vi "FL_Decode_RAW_to_DEC_bit_split_2b.vi"(2 "Read buffer text to decode":string, 3 "Input timestamp":timestamp, 4 "SB size (loc. var. only)":u8) -> (0 "DEC output cluster":T1)   [LabVIEW 2018, in "Tracker.lvlib"]
uses:
  Tracker.lvlib
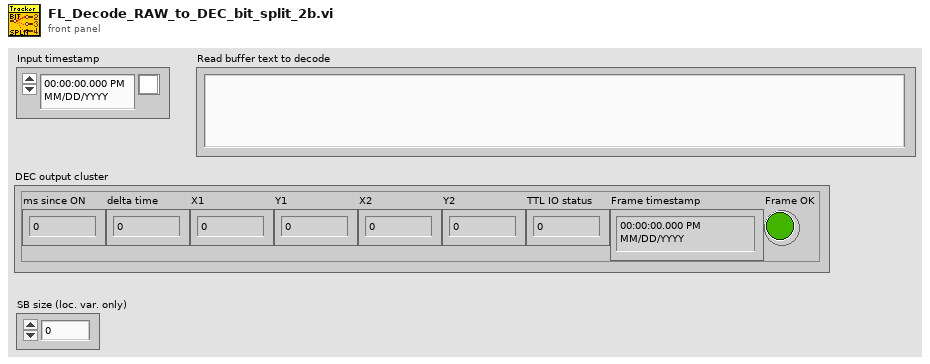
[diagram p1: front panel]
types:
  T1 = cluster{"ms since ON":u32, "delta time":u32, "X1":sgl, "Y1":sgl, "X2":sgl, "Y2":sgl, "TTL IO status":u8, "Frame timestamp":timestamp, "Frame OK":bool}
  T2 = cluster{"Half-width of the sensor board":sgl, "Half-height of the sensor board":sgl, "Sensors grid step":sgl}
  T3 = cluster{u32, u32, sgl, sgl, sgl, sgl, u8, "Input timestamp":timestamp, bool}
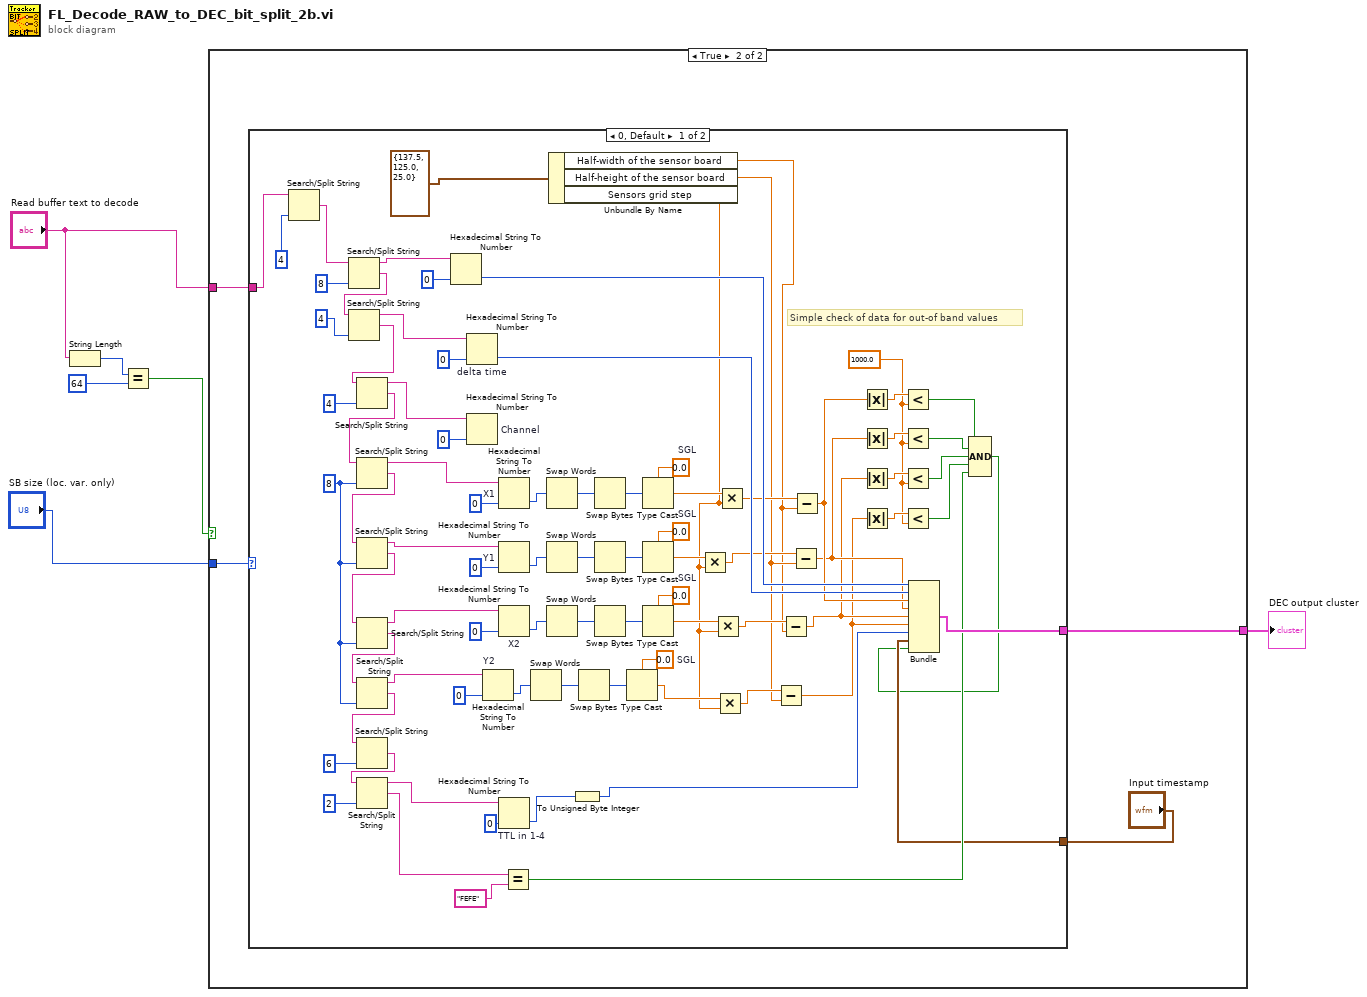
[diagram p0: block diagram]
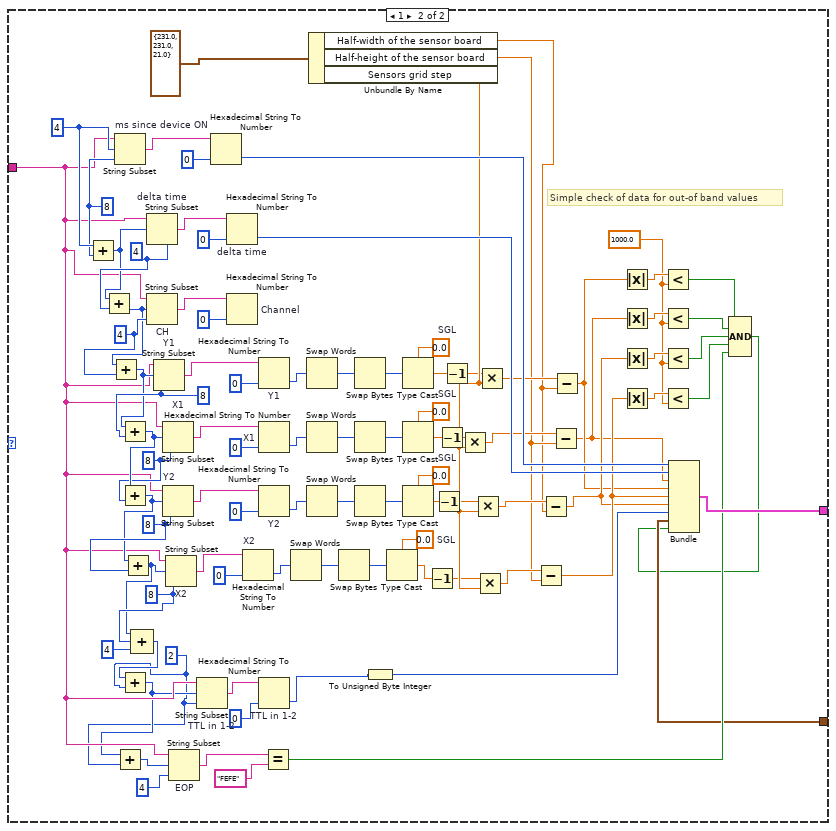
[diagram p3: hidden frame]
diagram:
  n1 = String Length(string="Read buffer text to decode") -> (length=w4:i32)
  n2 = Equal?(x=w4, y=64) -> (x = y?=w2:bool)
  n3 = case shown="True" w2 {
    tunnel: [_ w10] -> w6
    tunnel: "Read buffer text to decode" -> [_ w9]
    tunnel: "SB size (loc. var. only)" -> [_ w7]
    frame False {
    }
    frame True {
      n4 = case shown="0, Default" w7 {
        tunnel: [w60 w132] -> w10
        tunnel: w9 -> [w34 w129]
        tunnel: "Input timestamp" -> [w38 w104]
        frame 0, Default {
          w17 = 8 ("offset (0)")
          w50 = 1000.0
          w85 = sgl 0.0  # SGL
          w79 = sgl 0.0  # SGL
          w73 = sgl 0.0  # SGL
          w67 = sgl 0.0  # SGL
          # "Simple check of data for out-of band values"
          n5 = Search/Split String(string=w34, offset (0)=4) -> (match + rest of string=w36:string)  [unwired: 1 in, 2 out]
          n6 = Search/Split String(string=w36, offset (0)=8) -> (substring before match=w35:string, match + rest of string=w32:string)  [unwired: 1 in, 1 out]
          n7 = Search/Split String(string=w32, offset (0)=4 ("length (rest)")) -> (substring before match=w31:string, match + rest of string=w28:string)  [unwired: 1 in, 1 out]
          n8 = Search/Split String(string=w28, offset (0)=4) -> (substring before match=w27:string, match + rest of string=w25:string)  [unwired: 1 in, 1 out]
          n9 = Search/Split String(string=w25, offset (0)=w17) -> (substring before match=w21:string, match + rest of string=w24:string)  [unwired: 1 in, 1 out]
          n10 = Search/Split String(string=w24, offset (0)=w17) -> (substring before match=w20:string, match + rest of string=w23:string)  [unwired: 1 in, 1 out]
          n11 = Search/Split String(string=w23, offset (0)=w17) -> (substring before match=w19:string, match + rest of string=w22:string)  [unwired: 1 in, 1 out]
          n12 = Search/Split String(string=w22, offset (0)=w17) -> (substring before match=w18:string, match + rest of string=w16:string)  [unwired: 1 in, 1 out]
          n13 = Search/Split String(string=w16, offset (0)=6) -> (match + rest of string=w13:string)  [unwired: 1 in, 2 out]
          n14 = Search/Split String(string=w13, offset (0)=2) -> (substring before match=w12:string, match + rest of string=w11:string)  [unwired: 1 in, 1 out]
          n15 = Hexadecimal String To Number ("ms since ON")(string=w35, default (0uL)=u32 0 ("default (0 U32)")) -> (number=w94:u32)  [unwired: 1 in, 1 out]
          n16 = Hexadecimal String To Number "delta time"(string=w31, default (0uL)=u32 0 ("default (0 U32)")) -> (number=w93:u32)  [unwired: 1 in, 1 out]
          n17 = Hexadecimal String To Number "Channel"(string=w27, default (0uL)=u32 0 ("default (0 U32)")) -> ()  [unwired: 1 in, 2 out]
          n18 = Hexadecimal String To Number "Y2"(string=w18, default (0uL)=u32 0 ("default (0 U32)")) -> (number=w83:u32)  [unwired: 1 in, 1 out]
          n19 = Hexadecimal String To Number "X1"(string=w21, default (0uL)=u32 0 ("default (0 U32)")) -> (number=w65:u32)  [unwired: 1 in, 1 out]
          n20 = Hexadecimal String To Number "Y1"(string=w20, default (0uL)=u32 0 ("default (0 U32)")) -> (number=w71:u32)  [unwired: 1 in, 1 out]
          n21 = Hexadecimal String To Number "X2"(string=w19, default (0uL)=u32 0 ("default (0 U32)")) -> (number=w77:u32)  [unwired: 1 in, 1 out]
          n22 = Hexadecimal String To Number "TTL in 1-4"(string=w12, default (0uL)=u32 0 ("default (0 U32)")) -> (number=w40:u32)  [unwired: 1 in, 1 out]
          n23 = Equal?(x=w11, y="FEFE") -> (x = y?=w45:bool)
          n24 = Swap Words(1:w83) -> (0:w84:u32)
          n25 = Swap Words(1:w65) -> (0:w66:u32)
          n26 = Swap Words(1:w71) -> (0:w72:u32)
          n27 = Swap Words(1:w77) -> (0:w78:u32)
          n28 = Unbundle By Name(T2 {"Half-width of the sensor board"=137.5, "Half-height of the sensor board"=125.0, "Sensors grid step"=25.0} ("MHC geometry")) -> ("Half-width of the sensor board"=w42:sgl, "Half-height of the sensor board"=w43:sgl, "Sensors grid step"=w44:sgl)
          n29 = To Unsigned Byte Integer(number=w40) -> (unsigned 8bit integer=w39:u8)
          n30 = Swap Bytes(anything=w84) -> (byte swapped=w86:u32)
          n31 = Swap Bytes(anything=w66) -> (byte swapped=w68:u32)
          n32 = Swap Bytes(anything=w72) -> (byte swapped=w74:u32)
          n33 = Swap Bytes(anything=w78) -> (byte swapped=w80:u32)
          n34 = Type Cast(type=w85, x=w86) -> (*(type *) &x=w87:sgl)
          n35 = Type Cast(type=w67, x=w68) -> (*(type *) &x=w69:sgl)
          n36 = Type Cast(type=w73, x=w74) -> (*(type *) &x=w75:sgl)
          n37 = Type Cast(type=w79, x=w80) -> (*(type *) &x=w81:sgl)
          n38 = Multiply(x=w75, y=w44) -> (x*y=w90:sgl)
          n39 = Multiply(x=w81, y=w44) -> (x*y=w89:sgl)
          n40 = Multiply(x=w87, y=w44) -> (x*y=w91:sgl)
          n41 = Multiply(x=w69, y=w44) -> (x*y=w88:sgl)
          n42 = Subtract(x=w91, y=w43) -> (x-y=w55:sgl)
          n43 = Subtract(x=w89, y=w42) -> (x-y=w56:sgl)
          n44 = Subtract(x=w90, y=w43) -> (x-y=w57:sgl)
          n45 = Subtract(x=w88, y=w42) -> (x-y=w58:sgl)
          n46 = Absolute Value(x=w58) -> (abs(x)=w54:sgl)
          n47 = Absolute Value(x=w57) -> (abs(x)=w52:sgl)
          n48 = Absolute Value(x=w56) -> (abs(x)=w53:sgl)
          n49 = Absolute Value(x=w55) -> (abs(x)=w51:sgl)
          n50 = Less?(x=w54, y=w50) -> (x < y?=w49:bool)
          n51 = Less?(x=w52, y=w50) -> (x < y?=w48:bool)
          n52 = Less?(x=w53, y=w50) -> (x < y?=w47:bool)
          n53 = Less?(x=w51, y=w50) -> (x < y?=w46:bool)
          n54 = Compound Arithmetic op=AND(w49, w48, w47, w46, w45) -> (w37:bool)
          n55 = Bundle(w94, w93, w58, w57, w56, w55, w39, "Input timestamp"=w38, w37) -> (w60:T3)  [unwired: 1 in]
        }
        frame 1 {
          w120 = 1000.0
          w184 = 4
          w127 = 2 ("length (rest)")
          w171 = sgl 0.0  # SGL
          w165 = sgl 0.0  # SGL
          w159 = sgl 0.0  # SGL
          w154 = sgl 0.0  # SGL
          w179 = 8 ("length (rest)")
          w143 = 8 ("length (rest)")
          w140 = 8 ("length (rest)")
          w139 = 8 ("length (rest)")
          w137 = 4 ("length (rest)")
          w135 = 4 ("length (rest)")
          w133 = 8 ("length (rest)")
          # "Simple check of data for out-of band values"
          n56 = Add(x=w184, y=w133) -> (x+y=w134:i32)
          n57 = Add(x=w134, y=w135) -> (x+y=w136:i32)
          n58 = Add(x=w136, y=w137) -> (x+y=w138:i32)
          n59 = String Subset "ms since device ON"(string=w129, offset (0)=w184, length (rest)=w133) -> (substring=w144:string)
          n60 = Add(x=w138, y=w139) -> (x+y=w141:i32)
          n61 = Add(x=w141, y=w140) -> (x+y=w142:i32)
          n62 = Add(x=w142, y=w143) -> (x+y=w178:i32)
          n63 = Compound Arithmetic op=unknown(w178, w179, 4 ("value")) -> (w182:i32)
          n64 = Add(x=w182, y=w127) -> (x+y=w128:i32)
          n65 = Add(x=w128, y=w127) -> (x+y=w131:i32)
          n66 = String Subset "delta time"(string=w129, offset (0)=w134, length (rest)=w135) -> (substring=w147:string)
          n67 = String Subset "CH"(string=w129, offset (0)=w136, length (rest)=w137) -> (substring=w149:string)
          n68 = String Subset "Y1"(string=w129, offset (0)=w138, length (rest)=w139) -> (substring=w150:string)
          n69 = String Subset "X1"(string=w129, offset (0)=w141, length (rest)=w140) -> (substring=w161:string)
          n70 = String Subset "Y2"(string=w129, offset (0)=w142, length (rest)=w143) -> (substring=w167:string)
          n71 = String Subset "X2"(string=w129, offset (0)=w178, length (rest)=w179) -> (substring=w173:string)
          n72 = String Subset "EOP"(string=w129, offset (0)=w131, length (rest)=4 ("length (rest)")) -> (substring=w126:string)
          n73 = String Subset "TTL in 1-2"(string=w129, offset (0)=w128, length (rest)=w127) -> (substring=w180:string)
          n74 = Hexadecimal String To Number ("ms since ON")(string=w144, default (0uL)=u32 0 ("default (0 U32)")) -> (number=w186:u32)  [unwired: 1 in, 1 out]
          n75 = Hexadecimal String To Number "delta time"(string=w147, default (0uL)=u32 0 ("default (0 U32)")) -> (number=w185:u32)  [unwired: 1 in, 1 out]
          n76 = Hexadecimal String To Number "Channel"(string=w149, default (0uL)=u32 0 ("default (0 U32)")) -> ()  [unwired: 1 in, 2 out]
          n77 = Hexadecimal String To Number "X2"(string=w173, default (0uL)=u32 0 ("default (0 U32)")) -> (number=w169:u32)  [unwired: 1 in, 1 out]
          n78 = Hexadecimal String To Number "Y1"(string=w150, default (0uL)=u32 0 ("default (0 U32)")) -> (number=w152:u32)  [unwired: 1 in, 1 out]
          n79 = Hexadecimal String To Number "X1"(string=w161, default (0uL)=u32 0 ("default (0 U32)")) -> (number=w157:u32)  [unwired: 1 in, 1 out]
          n80 = Hexadecimal String To Number "Y2"(string=w167, default (0uL)=u32 0 ("default (0 U32)")) -> (number=w163:u32)  [unwired: 1 in, 1 out]
          n81 = Hexadecimal String To Number "TTL in 1-2"(string=w180, default (0uL)=u32 0 ("default (0 U32)")) -> (number=w106:u32)  [unwired: 1 in, 1 out]
          n82 = Equal?(x=w126, y="FEFE") -> (x = y?=w115:bool)
          n83 = Swap Words(1:w169) -> (0:w170:u32)
          n84 = Swap Words(1:w152) -> (0:w153:u32)
          n85 = Swap Words(1:w157) -> (0:w158:u32)
          n86 = Swap Words(1:w163) -> (0:w164:u32)
          n87 = Unbundle By Name(T2 {"Half-width of the sensor board"=231.0, "Half-height of the sensor board"=231.0, "Sensors grid step"=21.0} ("MHC geometry")) -> ("Half-width of the sensor board"=w112:sgl, "Half-height of the sensor board"=w113:sgl, "Sensors grid step"=w114:sgl)
          n88 = Swap Bytes(anything=w170) -> (byte swapped=w172:u32)
          n89 = Swap Bytes(anything=w153) -> (byte swapped=w155:u32)
          n90 = Swap Bytes(anything=w158) -> (byte swapped=w160:u32)
          n91 = Swap Bytes(anything=w164) -> (byte swapped=w166:u32)
          n92 = To Unsigned Byte Integer(number=w106) -> (unsigned 8bit integer=w105:u8)
          n93 = Type Cast(type=w171, x=w172) -> (*(type *) &x=w99:sgl)
          n94 = Type Cast(type=w154, x=w155) -> (*(type *) &x=w102:sgl)
          n95 = Type Cast(type=w159, x=w160) -> (*(type *) &x=w101:sgl)
          n96 = Type Cast(type=w165, x=w166) -> (*(type *) &x=w100:sgl)
          n97 = Decrement(x=w99) -> (x-1=w107:sgl)
          n98 = Decrement(x=w100) -> (x-1=w108:sgl)
          n99 = Decrement(x=w101) -> (x-1=w109:sgl)
          n100 = Decrement(x=w102) -> (x-1=w110:sgl)
          n101 = Multiply(x=w109, y=w114) -> (x*y=w176:sgl)
          n102 = Multiply(x=w108, y=w114) -> (x*y=w175:sgl)
          n103 = Multiply(x=w107, y=w114) -> (x*y=w177:sgl)
          n104 = Multiply(x=w110, y=w114) -> (x*y=w174:sgl)
          n105 = Subtract(x=w177, y=w113) -> (x-y=w98:sgl)
          n106 = Subtract(x=w175, y=w112) -> (x-y=w97:sgl)
          n107 = Subtract(x=w176, y=w113) -> (x-y=w95:sgl)
          n108 = Subtract(x=w174, y=w112) -> (x-y=w96:sgl)
          n109 = Absolute Value(x=w96) -> (abs(x)=w124:sgl)
          n110 = Absolute Value(x=w95) -> (abs(x)=w122:sgl)
          n111 = Absolute Value(x=w97) -> (abs(x)=w123:sgl)
          n112 = Absolute Value(x=w98) -> (abs(x)=w121:sgl)
          n113 = Less?(x=w124, y=w120) -> (x < y?=w119:bool)
          n114 = Less?(x=w122, y=w120) -> (x < y?=w118:bool)
          n115 = Less?(x=w123, y=w120) -> (x < y?=w117:bool)
          n116 = Less?(x=w121, y=w120) -> (x < y?=w116:bool)
          n117 = Compound Arithmetic op=AND(w119, w118, w117, w116, w115) -> (w103:bool)
          n118 = Bundle(w186, w185, w95, w96, w98, w97, w105, "Input timestamp"=w104, w103) -> (w132:T3)  [unwired: 1 in]
        }
      }
    }
  }
  "DEC output cluster" <- w6
